vi "DKr_2024.vi"(0 "Pressure / Pa":dbl=99951.0, 1 "xw mol fract water":dbl=0.013091, 2 "Frequency / Hz":dbl=20051.0, 3 "Temperature / K":dbl=293.4405 format="%.4g", 4 "CO2 content (ppm)":dbl=542.0, 5 "Type of air":i32(listbox)=4) -> (6 "DKr/1+Kr":dbl=2.1180286720406007e-05, 7 "DKr":dbl=2.118576028394063e-05 format="%.9f", 8 "Kr":dbl=0.0002584272633736037)   [LabVIEW 2016]
panel:
  out "fN2":dbl=4081.1365251244943
  out "fO2":dbl=4081.1365251244943 format="%_4g"
  out "DfO2":dbl=4081.1365251244943 format="%_4g"
  out "DfN2":dbl=55.66804727852973
  # "±"
  # "±"
  # "±"
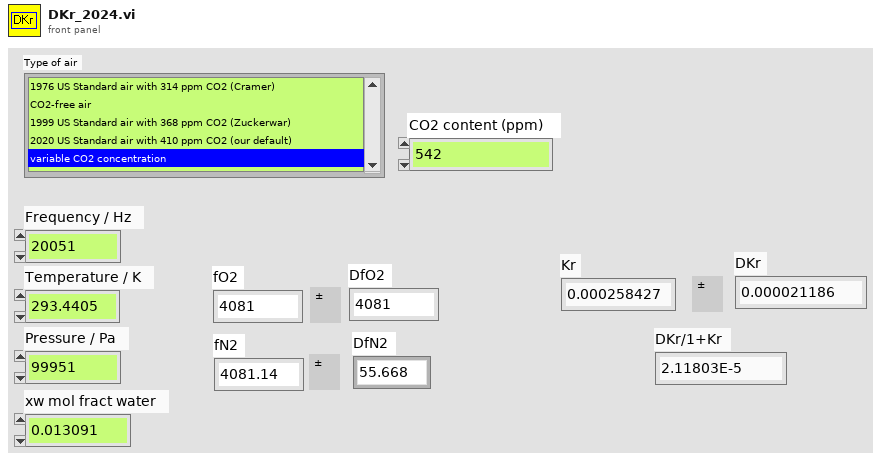
[diagram p1: front panel]
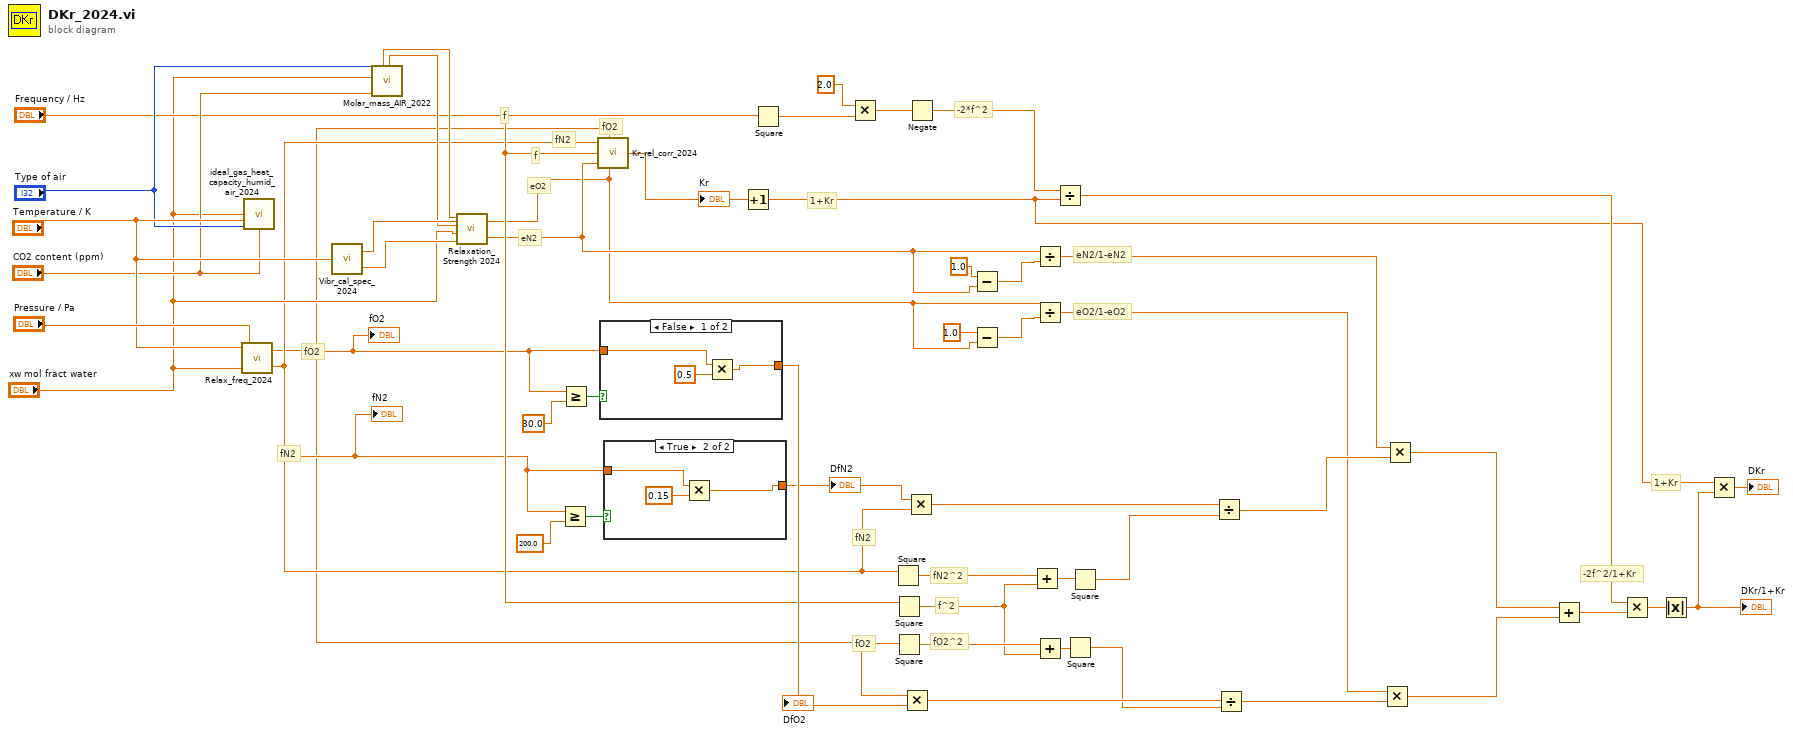
[diagram p0: block diagram]
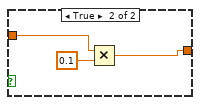
[diagram p2: hidden frame]
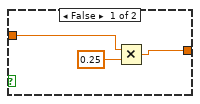
[diagram p3: hidden frame]
diagram:
  # "-2f^2/1+Kr"
  # "1+Kr"
  # "1+Kr"
  # "fO2"
  # "fO2^2"
  # "fN2"
  # "fN2^2"
  # "f^2"
  # "eO2/1-eO2"
  # "eN2/1-eN2"
  # "f"
  # "fO2"
  # "fN2"
  # "eO2"
  # "-2*f^2"
  # "f"
  # "fO2"
  # "fN2"
  # "eN2"
  n1 = call "Relax_freq_2024.vi"("H2O molar fraction"="xw mol fract water", "Pressure [Pa]"="Pressure / Pa", "Temperature [K]"="Temperature / K") -> ("Relax freq N2"=w2:dbl, "Relax freq O2"=w1:dbl)
  "fO2" <- w1
  "fN2" <- w2
  n2 = call "ideal_gas_heat_capacity_humid_air_2024.vi"("molar fraction of water vapor"="xw mol fract water", "Temperature [K]"="Temperature / K", "Type of air"="Type of air", "CO2 content (ppm)"="CO2 content (ppm)") -> ()  [unwired: 2 in, 10 out]
  n3 = call "Vibr_cal_spec_2024.vi"("Temperature [K]"="Temperature / K") -> ("Cvib O2 [J mol-1 K-1]"=w22:dbl, "Cvib N2 [J mol-1 K-1]"=w21:dbl)
  n4 = call "Molar_mass_AIR_2022.vi"("CO2 content (ppm)"="CO2 content (ppm)", "xw molar fraction of water vapor"="xw mol fract water", "Type of air"="Type of air") -> ("xN2"=w15:dbl, "xO2"=w16:dbl)  [unwired: 7 out]
  n5 = call "Relaxation_Strength 2024.vi"("C vib O2"=w22, "C vib N2"=w21, "xw molar fraction water vapor"="xw mol fract water", "N2 molar fraction Dry"=w15, "O2 molar fraction Dry"=w16) -> ("Rel strength N2"=w11:dbl, "Rel strength O2"=w10:dbl)  [unwired: 1 in]
  n6 = Greater Or Equal?(x=w2, y=200.0) -> (x >= y?=w27:bool)
  n7 = Greater Or Equal?(x=w1, y=30.0) -> (x >= y?=w25:bool)
  n8 = call "Kr_rel_corr_2024.vi"("N2 rel freq / Hz"=w2, "O2 rel freq / Hz"=w1, "Frequency / Hz"="Frequency / Hz", "N2 rel strength"=w11, "O2 rel strength"=w10) -> ("Kr"=w13:dbl)
  "Kr" <- w13
  n9 = case shown="False" w25 {
    tunnel: w1 -> [w52 w56]
    tunnel: [w51 w54] -> w23
    frame False {
      n10 = Multiply(x=w52, y=0.5) -> (x*y=w51:dbl)
    }
    frame True {
      n11 = Multiply(x=w56, y=0.1) -> (x*y=w54:dbl)
    }
  }
  "DfO2" <- w23
  n12 = case shown="True" w27 {
    tunnel: w2 -> [w58 w62]
    tunnel: [w57 w60] -> w12
    frame False {
      n13 = Multiply(x=w58, y=0.25) -> (x*y=w57:dbl)
    }
    frame True {
      n14 = Multiply(x=w62, y=0.15) -> (x*y=w60:dbl)
    }
  }
  "DfN2" <- w12
  n15 = Increment(x=w13) -> (x+1=w7:dbl)
  n16 = Square(x="Frequency / Hz") -> (x^2=w49:dbl)
  n17 = Multiply(x=2.0, y=w49) -> (x*y=w48:dbl)
  n18 = Square(x=w2) -> (x^2=w41:dbl)
  n19 = Square(x="Frequency / Hz") -> (x^2=w9:dbl)
  n20 = Square(x=w1) -> (x^2=w34:dbl)
  n21 = Multiply(x=w1, y=w23) -> (x*y=w36:dbl)
  n22 = Multiply(x=w12, y=w2) -> (x*y=w43:dbl)
  n23 = Negate(x=w48) -> (-x=w47:dbl)
  n24 = Subtract(x=1.0, y=w11) -> (x-y=w46:dbl)
  n25 = Subtract(x=1.0, y=w10) -> (x-y=w38:dbl)
  n26 = Add(x=w41, y=w9) -> (x+y=w40:dbl)
  n27 = Divide(x=w11, y=w46) -> (x/y=w44:dbl)
  n28 = Divide(x=w10, y=w38) -> (x/y=w8:dbl)
  n29 = Add(x=w34, y=w9) -> (x+y=w33:dbl)
  n30 = Divide(x=w47, y=w7) -> (x/y=w29:dbl)
  n31 = Square(x=w33) -> (x^2=w32:dbl)
  n32 = Square(x=w40) -> (x^2=w39:dbl)
  n33 = Divide(x=w43, y=w39) -> (x/y=w42:dbl)
  n34 = Divide(x=w36, y=w32) -> (x/y=w35:dbl)
  n35 = Multiply(x=w8, y=w35) -> (x*y=w30:dbl)
  n36 = Multiply(x=w44, y=w42) -> (x*y=w31:dbl)
  n37 = Add(x=w31, y=w30) -> (x+y=w28:dbl)
  n38 = Multiply(x=w29, y=w28) -> (x*y=w6:dbl)
  n39 = Absolute Value(x=w6) -> (abs(x)=w4:dbl)
  "DKr/1+Kr" <- w4
  n40 = Multiply(x=w7, y=w4) -> (x*y=→"DKr":dbl)
